vi "ScriptButton.vi"(9 "Priority":u8, 10 "Script Name":string, 11 "Button":bool) -> ()   [LabVIEW 2011]
uses:
  MutexMode.ctl
  <vilib>/Rock Robotics/WPI/DriverStation/WPI_DriverStationStatusErrorCache.ctl
  MutexState.ctl
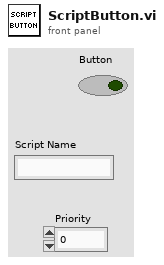
[diagram p1: front panel]
types:
  T1 = typedef "MutexState.ctl" = enum16{"Unlocked", "Locked-You", "Locked-Unknown", "Locked-ScriptButton", "Locked-Autonomous"}
  T2 = typedef "WPI_DriverStationStatusErrorCache.ctl" = enum16{"Get", "Set"}
  T3 = typedef "MutexMode.ctl" = enum16{"Get Mode", "Request Execution", "Stop Execution", "Lock Autonomous", "Script Completed"}
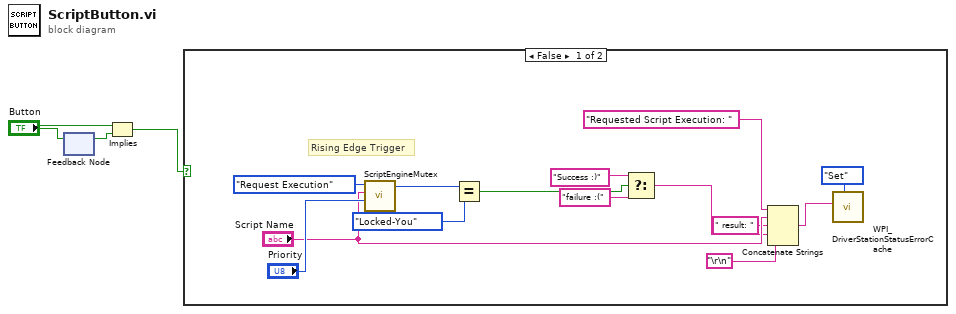
[diagram p0: block diagram]
diagram:
  n1 = feedback-in #1("Button") -> ()
  n2 = feedback #1() -> (w3:bool)  [unwired: 1 in]
  n3 = Implies(1:w3, 2:"Button") -> (0:w1:bool)
  n4 = case shown="False" w1 {
    frame False {
      # "Rising Edge Trigger"
      n5 = call "ScriptEngineMutex.vi"("Priority"="Priority", "Calling Script"="Script Name", "Mutex Mode"=MutexMode."Request Execution") -> ("Mutex State"=w9:T1)  [unwired: 8 in]
      n6 = Equal?(x=w9, y=MutexState."Locked-You") -> (x = y?=w7:bool)
      n7 = Select(t="Success :)", s=w7, f="failure :(") -> (s? t:f=w5:string)
      n8 = Concatenate Strings("Requested Script Execution: " ("string"), "Script Name", " result: " ("string"), w5, "\r\n") -> (w13:string)
      n9 = call <vilib>:"WPI_DriverStationStatusErrorCache.vi"("StatusErrorCacheOp"=WPI_DriverStationStatusErrorCache."Set", "Error String"=w13) -> ()  [unwired: 10 out]
    }
    frame True {
    }
  }
